vi "ACT_Test.vi"(0 "CurrentTest":T1 {"Post-Log(s)" format="%#_13g"; "Pre-Log (s)" format="%#_13g"; "Duration (s)" format="%#_13g"}, 1 "Path to Actuation Script":path=path "C:/Users/dpl/OneDrive - Aberystwyth University/Documents/Python/arguments/test.py", 2 "VideoSave Directory":path=path "E:/LTM Tests/VideoTests", 3 "Path to FFMPEG":path=path "C:/Program Files/FFMpeg/bin/ffmpeg.exe", 5 "DelayStr Ref":refnum<vi>, 9 "Test Prefix":string, 11 "error in (no error)":errorcluster, 12 "Video Camera":string="USB Camera", 13 "Actuation":i32, 14 "COM Port":i32) -> (8 "return code":i32, 15 "error out":errorcluster)   [LabVIEW 2025]
uses:
  controls/SingleTest.ctl
  controls/TestType.ctl
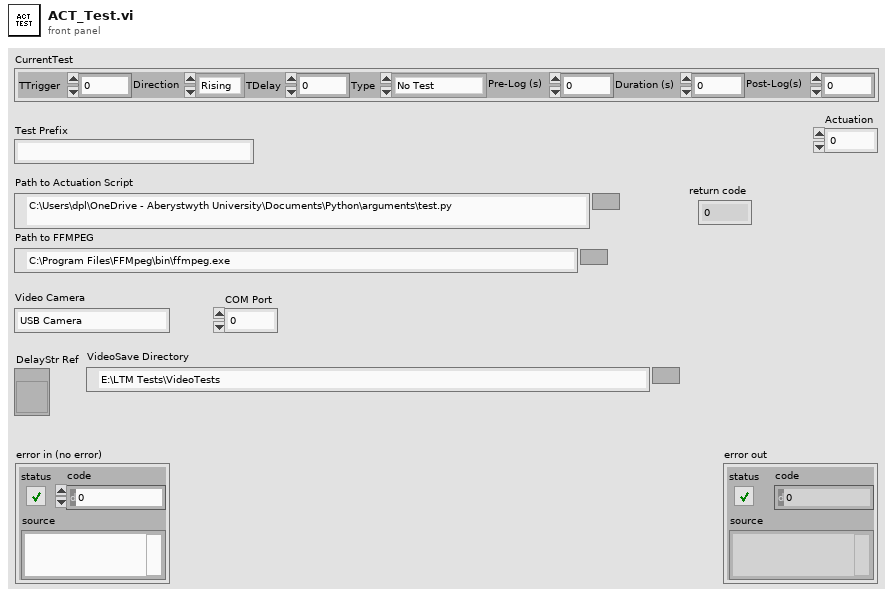
[diagram p1: front panel]
types:
  T1 = typedef "SingleTest.ctl" = cluster{"TTrigger":dbl, "Direction":enum16{"Rising", "Falling"}, "TDelay":dbl, "Type":T2, "Pre-Log (s)":dbl, "Duration (s)":dbl, "Post-Log(s)":dbl}
  T2 = typedef "TestType.ctl" = enum16{"No Test", "Heater Test", "Actuation Test", "Diode Test"}
  T3 = typedef "FFMpegRef.ctl" = cluster{"FFMpegRef":refnum<k24>, "StdOutRef":refnum<k24>, "DiagRef":refnum<k24>}
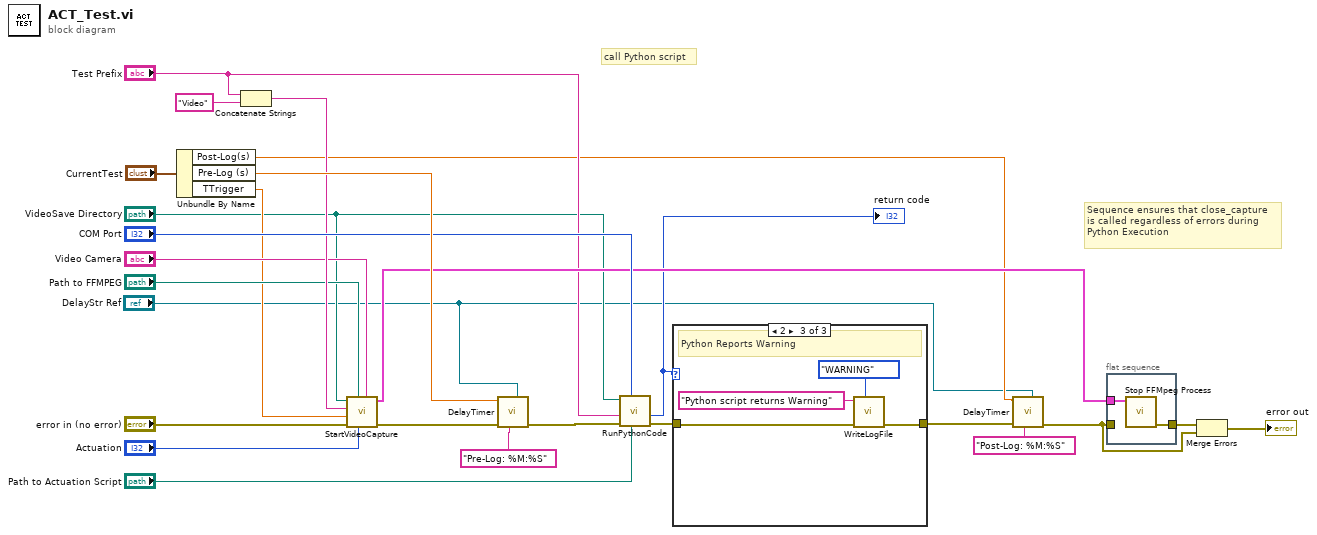
[diagram p0: block diagram]
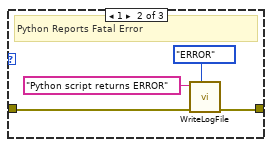
[diagram p3: hidden frame]
diagram:
  # "Sequence ensures that close_capture\nis called regardless of errors during \nPython Execution"
  # "call Python script"
  n1 = Unbundle By Name("CurrentTest") -> ("Post-Log(s)"=w14:dbl, "Pre-Log (s)"=w25:dbl, "TTrigger"=w6:dbl)
  n2 = Concatenate Strings("Test Prefix", "Video" ("string")) -> (w18:string)
  n3 = call "StartVideoCapture.vi"("Video Camera"="Video Camera", "Actuation"="Actuation", "Path to FFMPEG"="Path to FFMPEG", "error in (no error)"="error in (no error)", "TNom"=w6, "SaveFile"=w18, "Output Directory"="VideoSave Directory") -> ("error out"=w20:errorcluster, "FFMpegProcess"=w19:T3)  [unwired: 3 in]
  n4 = call "DelayTimer.vi"("Formatted \nTime Ref"="DelayStr Ref", "FormatString"="Pre-Log: %M:%S", "error in (no error)"=w20, "Delay(s)"=w25) -> ("error out"=w15:errorcluster)  [unwired: 7 in]
  n5 = call "RunPythonCode.vi"("Path to Actuation Script"="Path to Actuation Script", "COM Port"="COM Port", "error in (no error)"=w15, "TestPrefix"="Test Prefix", "Output base directory"="VideoSave Directory") -> ("error out"=w3:errorcluster, "return code"=w4:i32)  [unwired: 5 in]
  "return code" <- w4
  n6 = case shown="2" w4 {
    tunnel: w3 -> [w27 w30 w34]
    tunnel: [w27 w31 w35] -> w2
    frame 0, Default {
      # "No Errors"
    }
    frame 1 {
      # "Python Reports Fatal Error"
      n7 = call "WriteLogFile.vi"("Type"=enum16{"INFO", "WARNING", "ERROR"}."ERROR", "error in (no error)"=w30, "Message"="Python script returns ERROR") -> ("error out"=w31:errorcluster)  [unwired: 8 in]
    }
    frame 2 {
      # "Python Reports Warning"
      n8 = call "WriteLogFile.vi"("Type"=enum16{"INFO", "WARNING", "ERROR"}."WARNING", "error in (no error)"=w34, "Message"="Python script returns Warning") -> ("error out"=w35:errorcluster)  [unwired: 8 in]
    }
  }
  n9 = call "DelayTimer.vi"("Formatted \nTime Ref"="DelayStr Ref", "FormatString"="Post-Log: %M:%S", "error in (no error)"=w2, "Delay(s)"=w14) -> ("error out"=w9:errorcluster)  [unwired: 7 in]
  n10 = flat-sequence {
    tunnel: w19 -> [w37]
    tunnel: w9 -> [_]
    tunnel: [w36] -> w10
    frame #0 {
      n11 = call "Stop FFMpeg Process.vi"("FFMpegProcess"=w37) -> ("error out"=w36:errorcluster)  [unwired: 10 in]
    }
  }
  n12 = Merge Errors(w10, w9) -> (→"error out":errorcluster)
